vi "CSM-MassData Cache Status Viewer.vi"() -> ()   [LabVIEW 2017]
doc: "CSM Massdata cache status viewing tool that allows for an intuitive view of Massdata cache usage, helping to debug and optimize cache configuration.\n\n\n> [!NOTE] <b>CSM Massdata Argument Support</b>\n>\n> CSM Massdata argument support provides an efficient argument passing mechanism for transferring large amounts of data within CSM. By using a memory-efficient reference mechanism instead of direct data transfer, CSM Massdata improves the efficiency and performance of argument passing.\n> - The argument type defined by CSM Massdata is `<MassData>`, which can be obtained using the CSM - Argument Type VI.\n> - Data transmission of CSM Massdata is completely lossless. However, it is not suitable for storing data that requires indefinite persistence.\n>\n> <b>Note</b>: CSM Massdata internally uses a circular buffer mechanism. All CSM modules within the same application share the same Massdata buffer space. When the buffer is full, new data will overwrite old data starting from the beginning. Therefore, you need to set a reasonable buffer size to ensure that data is not overwritten before use, avoiding data loss."
uses:
  addons/MassData-Parameter/_support/FGV-MassData(lvlibp).vi
  addons/MassData-Parameter/CSM MassData Parameter Support.lvlib
  <userlib>/_NEVSTOP/Communicable State Machine(CSM)/_tool/_ui/csm-ui-support.lvlib
panel:
  in  "CacheSize(Byte)":u32 format="%.0p"
  in  "Remove all Configurations":bool
  out "Write":cluster{dbl, dbl}(slide)={287840.0, 276144.0} scale=1.0..50000000.0 scale format="%#_6p"
  out "Read":cluster{dbl, dbl}(slide)={287840.0, 276144.0} scale=1.0..50000000.0 scale format="%#_6p"
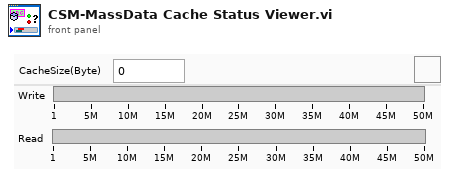
[diagram p1: front panel]
types:
  T1 = typedef "CSM MassData Parameter Support.lvlib/Def-MassDataOper-Status.ctl" = cluster{"Start":i32, "Size":i32, "Total":i32}
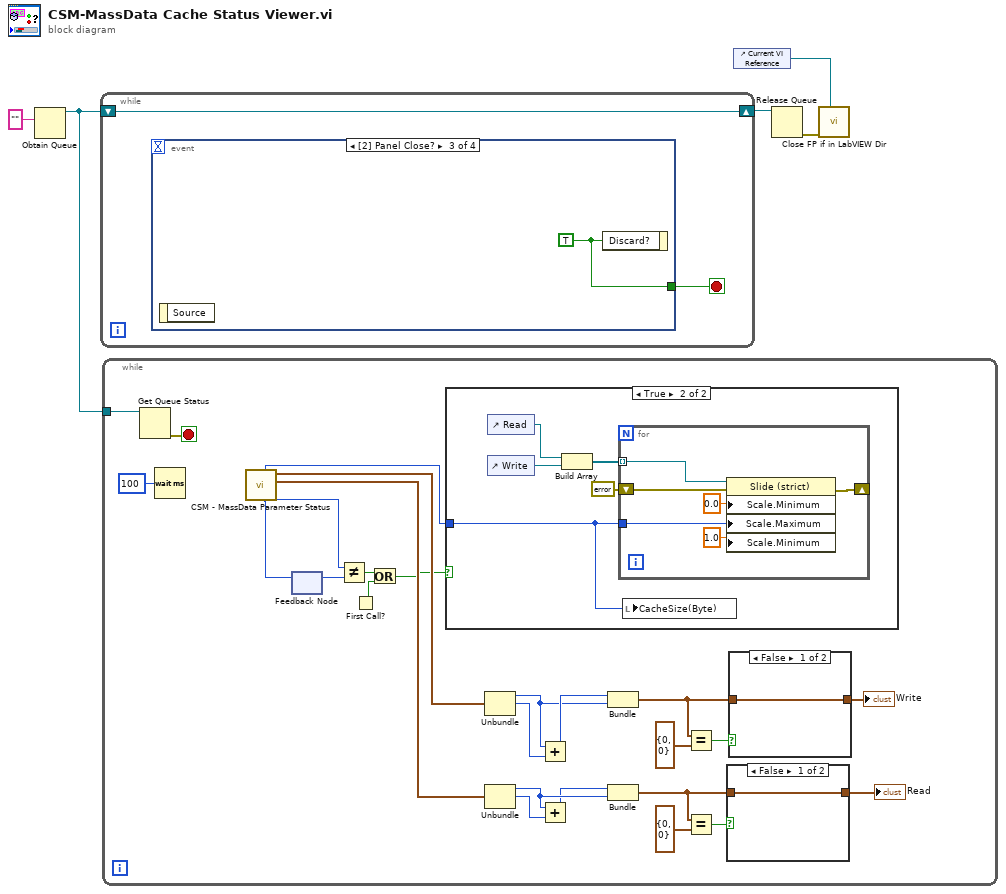
[diagram p0: block diagram]
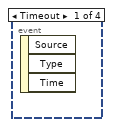
[diagram p2: hidden frame]
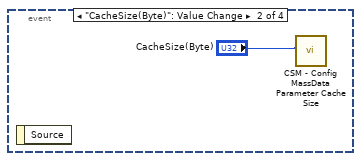
[diagram p3: hidden frame]
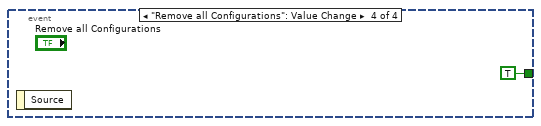
[diagram p4: hidden frame]
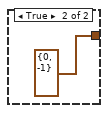
[diagram p5: hidden frame]
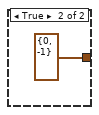
[diagram p6: hidden frame]
diagram:
  n1 = Obtain Queue(element data type="" ("name (unnamed)")) -> (queue out=w5:refnum<queue>)  [unwired: 4 in, 2 out]
  n2 = while {
    shift-right: [w6] -> w4
    shift-left: w5 -> [w6]
    stop <- w7 stop-if-true
    n3 = event shown="[2] Panel Close?" {
      selector: _ -> [_ _ _ _]
      dyn-events: _ -> [_ _ _ _]
      timeout: _ -> [_ _ _ _]
      tunnel: [_ _ w9 TRUE ("Discard?")] -> w7
      event Timeout {
        n4 = event-data() -> ()  [unwired: 1 in, 3 out]
      }
      event "CacheSize(Byte)": Value Change {
        n5 = event-data() -> ()  [unwired: 1 in, 1 out]
        n6 = call "CSM - Config MassData Parameter Cache Size.vi"("Size (50M)"="CacheSize(Byte)") -> ()  [unwired: 10 in, 1 out]
      }
      event Panel Close? {
        w9 = TRUE ("Discard?")
        n7 = event-data() -> ()  [unwired: 1 in, 1 out]
        n8 = event-data("Discard?"=w9) -> ()  [unwired: 1 in, 1 out]
      }
      event "Remove all Configurations": Value Change {
        n9 = event-data() -> ()  [unwired: 1 in, 1 out]
      }
    }
  }
  n10 = while {
    tunnel: w5 -> [w32]
    stop <- w33 stop-if-true
    n11 = Get Queue Status(queue=w32) -> (error out=w33:errorcluster)  [unwired: 2 in, 7 out]
    n12 = Wait (ms)(milliseconds to wait=u32 100) -> ()  [unwired: 1 out]
    n13 = call "CSM - MassData Parameter Status.vi"() -> ("Active Read Operation"=w30:T1, "Active Write Operation"=w31:T1, "Cache Size"=w21:i32)  [unwired: 7 in, 1 out]
    n14 = feedback #1() -> (w22:i32)  [unwired: 1 in]
    n15 = feedback-in #1(w21) -> ()
    n16 = Not Equal?(x=w21, y=w22) -> (x != y?=w23:bool)
    n17 = First Call?() -> (First Call?: T/F=w19:bool)
    n18 = Or(x=w23, y=w19) -> (x .or. y?=w20:bool)
    n19 = case shown="True" w20 {
      tunnel: w21 -> [_ w40]
      frame False {
      }
      frame True {
        n20 = control-ref of="Read"() -> (w43:refnum<vi>)
        n21 = control-ref of="Write"() -> (w42:refnum<vi>)
        n22 = Build Array(w43, w42) -> (w41:refnum<vi>[])
        n23 = for {
          tunnel: w40 -> [w49]
          shift-right: [w46] -> _
          shift-left: errorcluster {"status"=FALSE, "code"=0, "source"=""} ("error out") -> [w45]
          tunnel: w41 -> [w44] mode=indexing
          n24 = property on="Property Node" class="Slide (strict)"(reference=w44, error in=w45, "Scale.Minimum"=0.0 ("Scale.Range:Minimum"), "Scale.Maximum"=w49, "Scale.Minimum"=1.0 ("Scale.Range:Minimum")) -> (error out=w46:errorcluster)  [unwired: 1 out]
        }
        n25 = local write "CacheSize(Byte)"(w40) -> ()
      }
    }
    n26 = Unbundle(w31) -> ("Start"=w13:i32, "Size"=w15:i32)  [unwired: 1 out]
    n27 = Unbundle(w30) -> ("Start"=w18:i32, "Size"=w16:i32)  [unwired: 1 out]
    n28 = Add(x=w13, y=w15) -> (x+y=w14:i32)
    n29 = Add(x=w18, y=w16) -> (x+y=w17:i32)
    n30 = Bundle(w14, "Start"=w13) -> (w27:cluster{i32, "Start":i32})  [unwired: 1 in]
    n31 = Bundle(w17, "Start"=w18) -> (w26:cluster{i32, "Start":i32})  [unwired: 1 in]
    n32 = Equal?(x=w27, y=cluster{i32, "Start":i32} {0, "Start"=0}) -> (x = y?=w24:bool)
    n33 = Equal?(x=w26, y=cluster{i32, "Start":i32} {0, "Start"=0}) -> (x = y?=w25:bool)
    n34 = case shown="False" w25 {
      tunnel: w26 -> [w35 _]
      tunnel: [w35 cluster{i32, "Start":i32} {0, "Start"=-1}] -> w29
      frame False {
      }
      frame True {
      }
    }
    "Read" <- w29
    n35 = case shown="False" w24 {
      tunnel: [w37 cluster{i32, "Start":i32} {0, "Start"=-1}] -> w28
      tunnel: w27 -> [w37 _]
      frame False {
      }
      frame True {
      }
    }
    "Write" <- w28
  }
  n36 = control-ref of="Current VI Reference"() -> (w1:refnum<vi>)
  n37 = Release Queue(queue=w4) -> (error out=w2:errorcluster)  [unwired: 2 in, 2 out]
  n38 = call <userlib>:"Close FP if in LabVIEW Dir.vi"("VI Refnum"=w1, "Error in"=w2) -> ()  [unwired: 9 in, 1 out]
